vi "Write Emergency.vi"(8 "error in (no error)":errorcluster, 10 "Emergency Button":bool, 11 "User Console in":refnum<class "User Console.lvclass">) -> (0 "error out":errorcluster, 3 "User Console out":refnum<class "User Console.lvclass">)   [LabVIEW 2019, in "User Console Actor.lvlib" / "User Console.lvclass"]
uses:
  User Console.lvclass
  User Console.lvclass/User Console.ctl
  Abstract User Console Actor/Abstract User Console Actor/Abstract User Console.lvclass
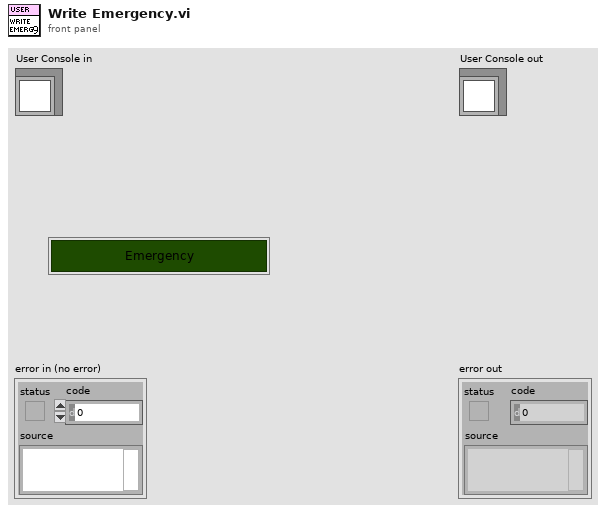
[diagram p1: front panel]
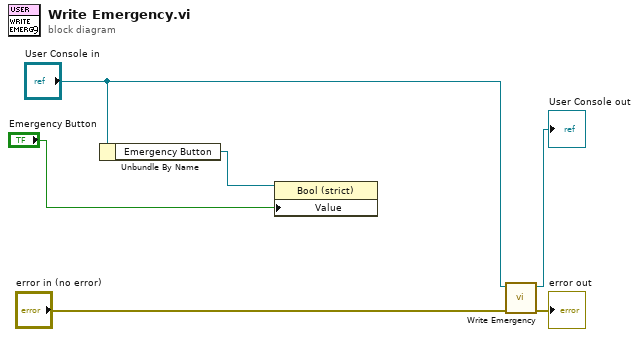
[diagram p0: block diagram]
diagram:
  n1 = Unbundle By Name("User Console in") -> ("Emergency Button"=w2:refnum<vi>)
  n2 = property class="Bool (strict)"(reference=w2, "Value"="Emergency Button") -> ()  [unwired: 1 in, 2 out]
  n3 = call-parent "Write Emergency.vi"("error in (no error)"="error in (no error)", "Abstract User Console in"="User Console in") -> ("error out"=→"error out":errorcluster, "Abstract User Console out"=→"User Console out":refnum<class "User Console.lvclass">)  [unwired: 8 in]
